vi "Z Aux Direct Move Spiral.vi"(0 "handle":u32, 1 "pitch":sgl, 2 "distance4":sgl, 5 "centre1":sgl, 7 "centre2":sgl, 9 "circles":sgl, 11 "error in (no error)":errorcluster caption="错误输入（无错误）", 12 "distance3":sgl) -> (4 "handle out":u32, 6 "function return":i32, 15 "error out":errorcluster caption="错误输出")   [LabVIEW 2015, in "zauxdll.lvlib"]
doc: "int32 __stdcall ZAux_Direct_MoveSpiral(ZMC_HANDLE handle, float centre1, float centre2, float circles, float pitch, float distance3, float distance4);"
uses:
  zauxdll.lvlib
  zauxdll.dll
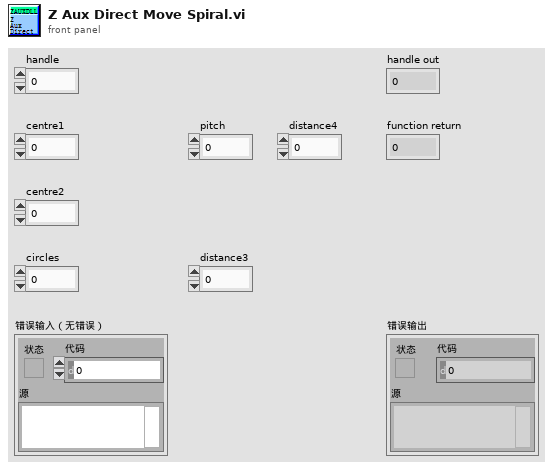
[diagram p1: front panel]
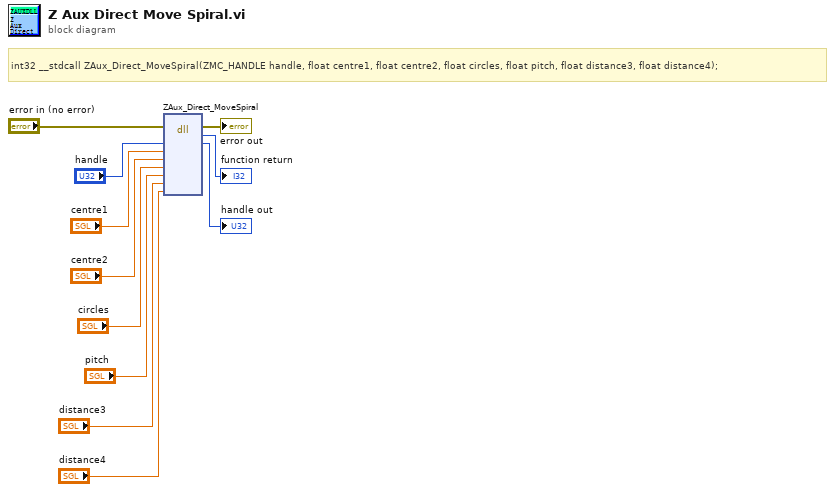
[diagram p0: block diagram]
diagram:
  # "int32 __stdcall ZAux_Direct_MoveSpiral(ZMC_HANDLE handle, float centre1, float centre2, float circles, float pitch, float distance3, float distance4);"
  n1 = dll-call lib="C:/Users/VIC/Desktop/GOGORO_Oringnal - Panasonic/system/LLB/zmotion/zaux/zauxdll.*" fn="ZAux_Direct_MoveSpiral"(error in="error in (no error)", "handle"="handle", "centre1"="centre1", "centre2"="centre2", "circles"="circles", "pitch"="pitch", "distance3"="distance3", "distance4"="distance4") -> (error out=→"error out":errorcluster, →"function return":i32, "handle"=→"handle out":u32)  [unwired: 8 in, 1 out]
